vi "Gate Delay Control.vi"(7 "Calling VI Ref":refnum<vi>) -> ()   [LabVIEW 2016]
uses:
  Gate Delay Type Defs/Delay Control.ctl
  <vilib>/Utility/miscctls.llb/LVPointTypeDef.ctl
  <vilib>/event_ctls.llb/lveventtype.ctl
  Gate Delay Type Defs/Board Names.ctl
  Gate Delay Type Defs/Gate Delay Actions.ctl
panel:
  in  "Link":bool
  in  "Restore Defaults":bool
  in  "Set Defaults":bool
  in  "Board Selection":enum32{"Delay 01", "Delay 02"}(radio)
  in  "Window Width":T1 {"Delay Slider" scale=0.0..9.5; "Delay (ns)" format="%#_4g"}
  in  "Window Delay":T1 {"Delay Slider" scale=0.0..19.5; "Delay (ns)" format="%#_4g"}
  in  "Laser Delay":T1 {"Delay Slider" scale=0.0..19.5; "Delay (ns)" format="%#_4g"}
  in  "Quit":bool
  # "Delay (ns)"
  # "Step (ns)"
  # "Window Width"
  # "Window Delay"
  # "Laser Delay"
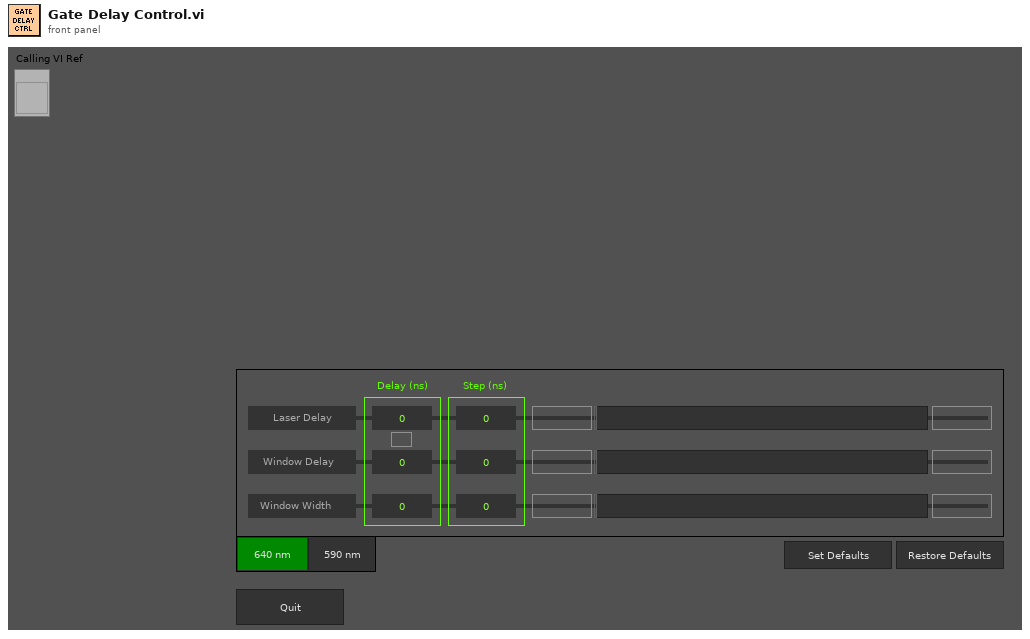
[diagram p1: front panel]
types:
  T1 = typedef "Delay Control.ctl" = cluster{"Delay (ns)":dbl, "Step (ns)":dbl, "Step Minus":bool, "Delay Slider":dbl, "Step Plus":bool}
  T2 = enum16{"Always On", "Always Off", "Off While Running"}
  T3 = typedef "LVPointTypeDef.ctl" = cluster{"Horizontal":i16, "Vertical":i16}
  T4 = typedef "lveventtype.ctl" = enum32{"Null", "Timeout", "Annotation Menu Selection", "Annotation Menu Selection?", "App Instance Close", "App Instance Close?", "Autoscale Range Change", "Bookmark Info Change", "Cell Edit", "Cell Edit?", "Cursor Grab", "Cursor Grab?", "Cursor Menu Selection", "Cursor Menu Selection?", "Cursor Move", "Cursor Release", "Data Change", "Direction Change", "Display State Change", "Drag Ended", "Drag Enter", "Drag Leave", "Drag Over", "Drag Source Update", "Drag Starting", "Drag Starting?", "Drop", "Exec State Change", "Key Down", "Key Down?", "Key Repeat", "Key Repeat?", "Key Up", "Listbox Double Click", "Menu Activation?", "Menu Selection (App)", "Menu Selection? (App)", "Menu Selection (User)", "Mouse Down", "Mouse Down?", "Mouse Enter", "Mouse Leave", "Mouse Move", "Mouse Up", "Mouse Wheel", "NI Security User Change (App)", "Pane Size", "Panel Close", "Panel Close?", "Panel Resize", "Plot Attribute Change", "Scale Range Change", "Shortcut Menu Activation?", "Shortcut Menu Selection (App)", "Shortcut Menu Selection? (App)", "Shortcut Menu Selection (User)", "Tree Double Click", "Tree Drag", "Tree Drag?", "Tree Drop", "Tree Drop?", "Tree Item Close", "Tree Item Close?", "Tree Item Open", "Tree Item Open?", "User Event", "Value Change"}
  T5 = typedef "Gate Delay Actions.ctl" = enum16{"Set Laser Delay", "Set Window Delay", "Set Window Width", "Get Delays", "Set Default Delays", "Restore Defaults", "Quit"}
  T6 = typedef "Board Names.ctl" = enum16{"Gate Delay 01", "Gate Delay 02"}
  T7 = enum32{"Bad", "Idle", "Run top level", "Running"}
  T8 = typedef "LVRectTypeDef.ctl" = cluster{"Left":i16, "Top":i16, "Right":i16, "Bottom":i16}
  T9 = typedef "LVBoundsTypeDef.ctl" = cluster{"Width":u32, "Height":u32}
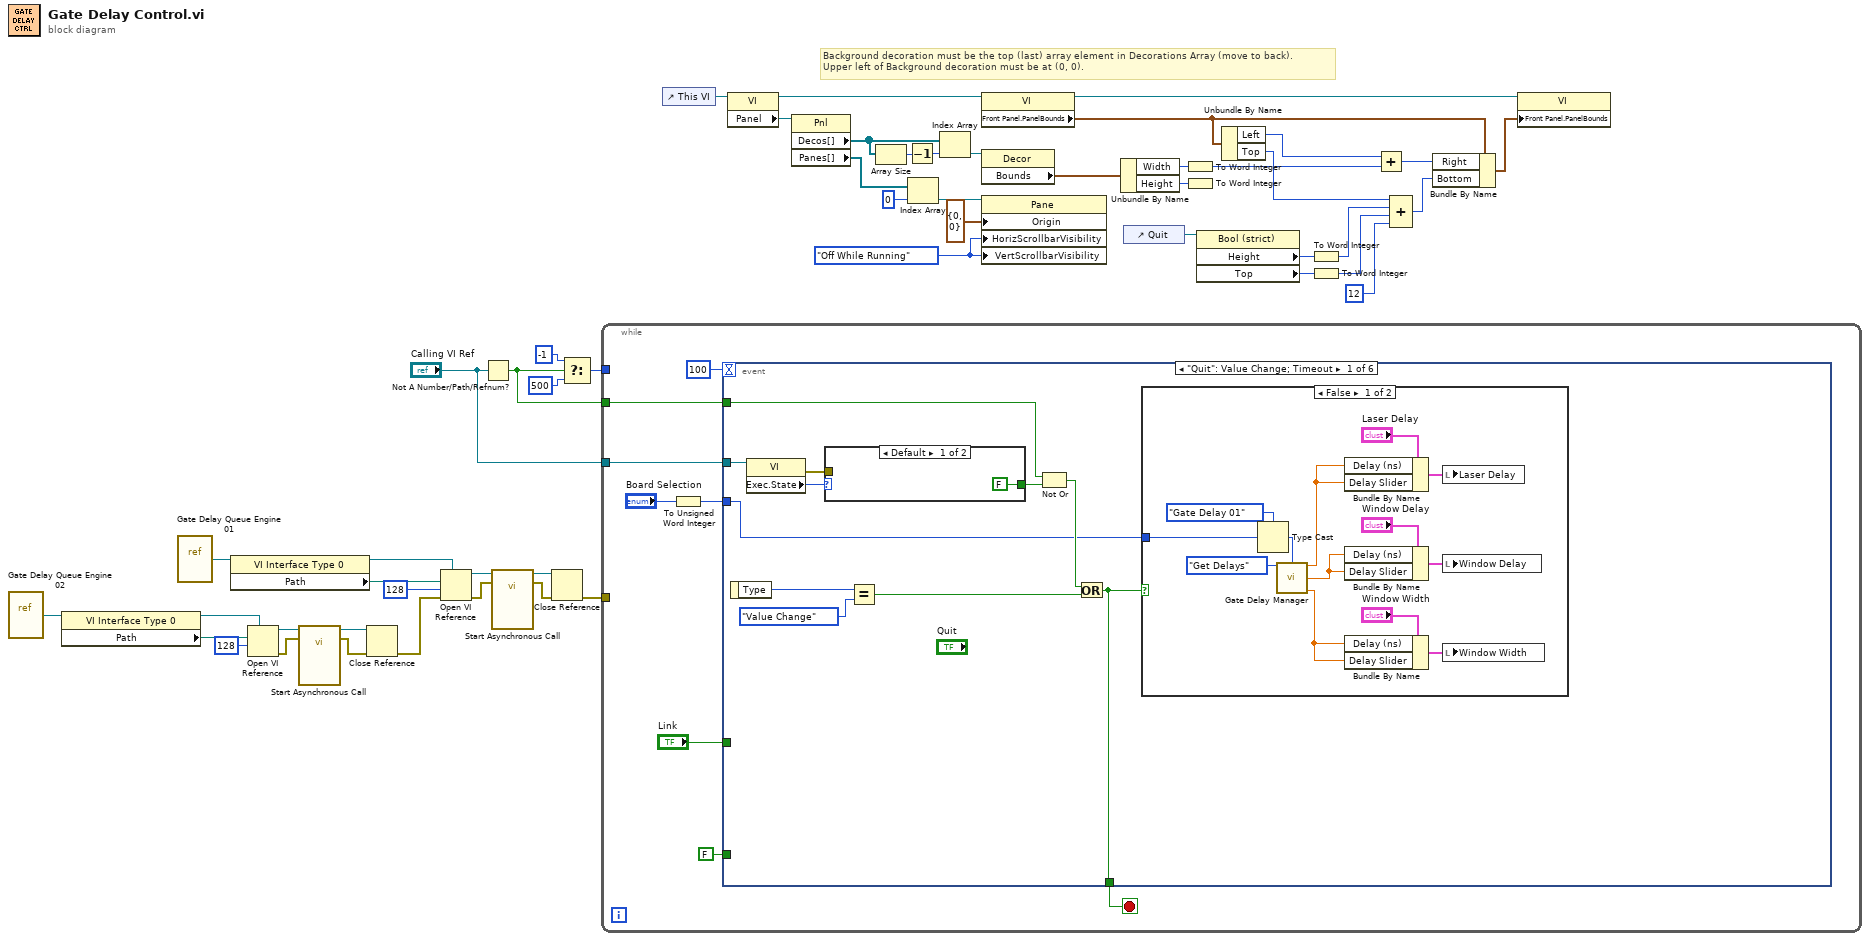
[diagram p0: block diagram]
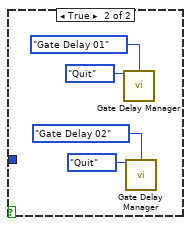
[diagram p2: hidden frame]
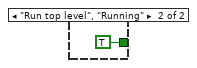
[diagram p3: hidden frame]
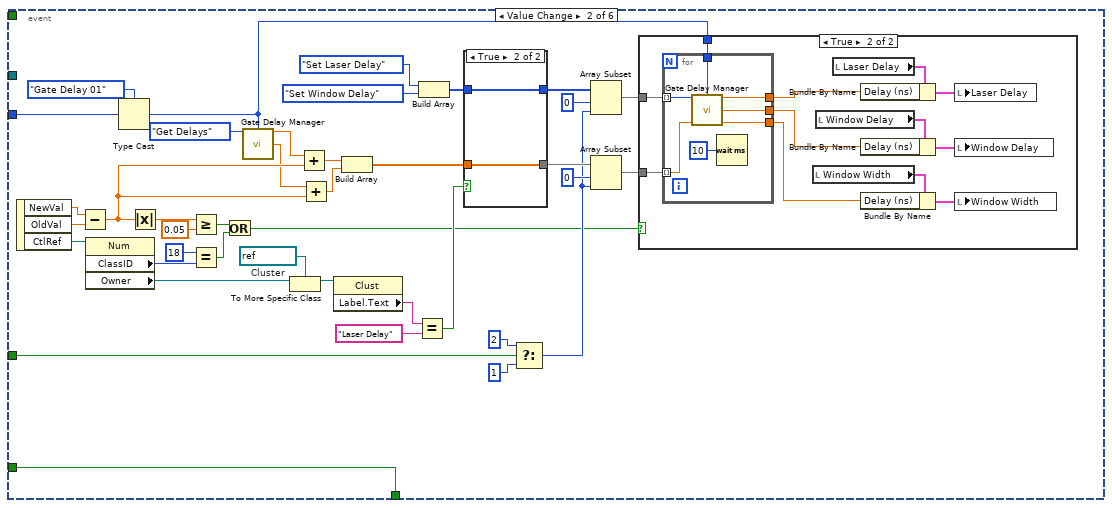
[diagram p4: hidden frame]
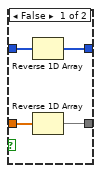
[diagram p6: hidden frame]
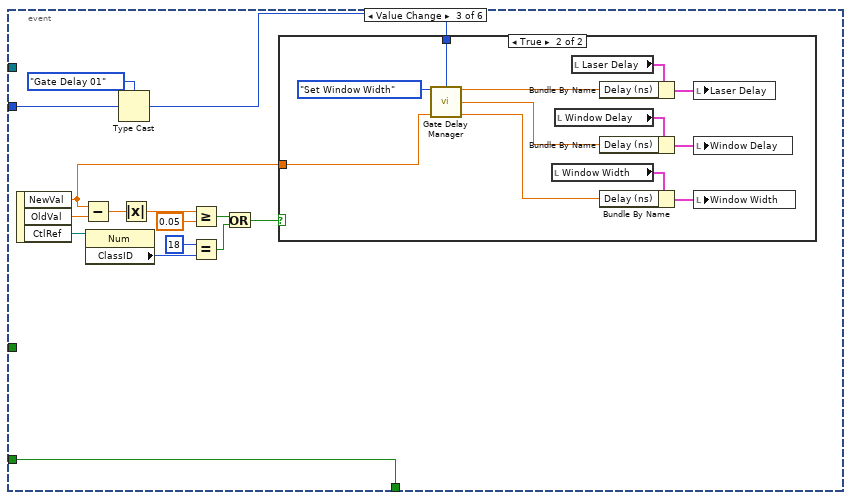
[diagram p7: hidden frame]
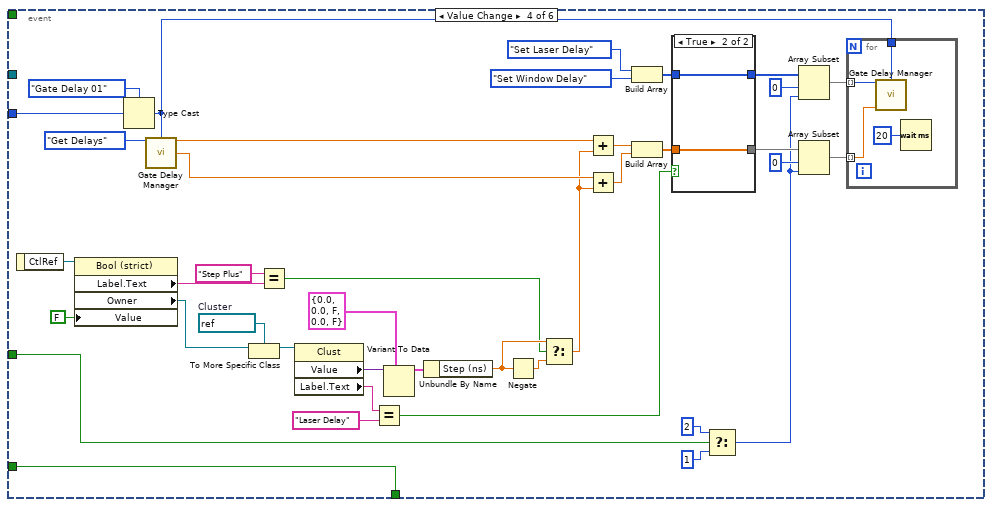
[diagram p9: hidden frame]
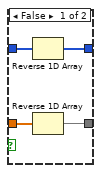
[diagram p10: hidden frame]
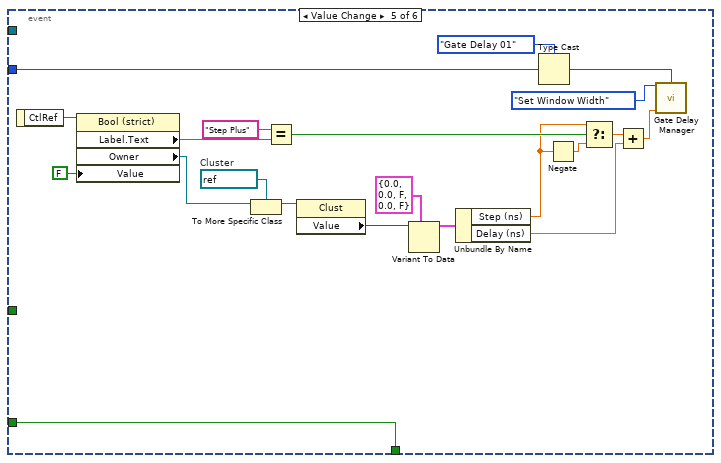
[diagram p11: hidden frame]
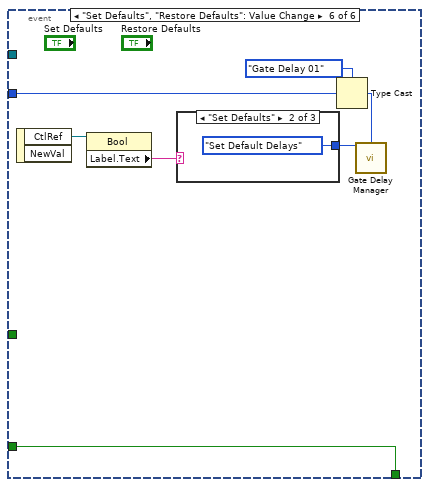
[diagram p12: hidden frame]
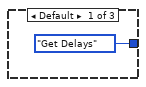
[diagram p13: hidden frame]
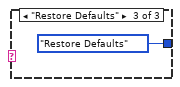
[diagram p14: hidden frame]
diagram:
  w30 = T2."Off While Running" ("Vertical Scrollbar Visibility")
  # "Background decoration must be the top (last) array element in Decorations Array (move to back).\nUpper left of Background decoration must be at (0, 0)."
  n1 = vi-ref "Gate Delay Queue Engine 02.vi"() -> (w11:refnum<vi>)
  n2 = property class="VI Interface Type 0"(reference=w11) -> (reference out=w9:refnum<vi>, "Path"=w10:path)  [unwired: 1 in, 1 out]
  n3 = vi-ref "Gate Delay Queue Engine 01.vi"() -> (w17:refnum<vi>)
  n4 = property class="VI Interface Type 0"(reference=w17) -> (reference out=w15:refnum<vi>, "Path"=w16:path)  [unwired: 1 in, 1 out]
  n5 = Open VI Reference(type specifier VI Refnum (for type only)=w9, vi path=w10, options=128) -> (vi reference=w8:refnum<vi>, error out=w6:errorcluster)  [unwired: 3 in]
  n6 = call-by-ref "Start Asynchronous Call"(reference=w8, error in=w6) -> (reference out=w7:refnum<vi>, error out=w5:errorcluster)  [unwired: 12 in]
  n7 = Close Reference(reference=w7, error in (no error)=w5) -> (error out=w4:errorcluster)
  n8 = Open VI Reference(type specifier VI Refnum (for type only)=w15, vi path=w16, options=128, error in (no error)=w4) -> (vi reference=w14:refnum<vi>, error out=w3:errorcluster)  [unwired: 2 in]
  n9 = Not A Number/Path/Refnum?(number/path/refnum="Calling VI Ref") -> (NaN/Path/Refnum?=w48:bool)
  n10 = call-by-ref "Start Asynchronous Call"(reference=w14, error in=w3) -> (reference out=w13:refnum<vi>, error out=w2:errorcluster)  [unwired: 12 in]
  n11 = Close Reference(reference=w13, error in (no error)=w2) -> (error out=w1:errorcluster)
  n12 = Select(t=-1, s=w48, f=500) -> (s? t:f=w50:i32)
  n13 = while {
    tunnel: w50 -> [_]
    tunnel: "Calling VI Ref" -> [w58]
    tunnel: w48 -> [w57]
    tunnel: w1 -> [_]
    stop <- w60 stop-if-true
    n14 = To Unsigned Word Integer(number="Board Selection") -> (unsigned 16bit integer=w55:u16)
    n15 = event shown="[0] \"Quit\": Value Change;  Timeout" {
      selector: _ -> [_ _ _ _ _ _]
      dyn-events: _ -> [_ _ _ _ _ _]
      timeout: 100 -> [_ _ _ _ _ _]
      tunnel: [w62 w130 w170 w222 w253 w260] -> w60
      tunnel: FALSE ("NewVal") -> [_ w130 w170 w222 w253 w260]
      tunnel: w58 -> [w71 _ _ _ _ _]
      tunnel: w57 -> [w66 _ _ _ _ _]
      tunnel: w55 -> [w61 w116 w160 w213 w240 w255]
      tunnel: "Link" -> [_ w100 _ w188 _ _]
      event "Quit": Value Change; Timeout {
        n16 = event-data() -> ("Type"=w69:T4)  [unwired: 1 in]
        n17 = property class="VI"(reference=w71) -> (error out=w63:errorcluster, "Exec.State"=w70:T7)  [unwired: 1 in, 1 out]
        n18 = case shown="Default" w70 {
          tunnel: [FALSE TRUE] -> w65
          tunnel: w63 -> [_ _]
          frame Default {
          }
          frame "Run top level", "Running" {
          }
        }
        n19 = Equal?(x=w69, y=lveventtype."Value Change" ("Type")) -> (x = y?=w67:bool)
        n20 = Not Or(1:w65, 2:w66) -> (0:w64:bool)
        n21 = Or(x=w64, y=w67) -> (x .or. y?=w62:bool)
        n22 = case shown="False" w62 {
          tunnel: w61 -> [w72 _]
          frame False {
            n23 = Type Cast(type=Board_Names."Gate Delay 01" ("Gate Delay Names"), x=w72) -> (*(type *) &x=w84:T6)
            n24 = call "Gate Delay Manager.vi"("Gate Delay Actions"=Gate_Delay_Actions."Get Delays", "Gate Delay Names"=w84) -> ("Laser Delay (ns)"=w74:dbl, "Window Delay (ns)"=w75:dbl, "Window Width (ns)"=w73:dbl)  [unwired: 11 in]
            n25 = Bundle By Name(cluster="Laser Delay", "Delay (ns)"=w74, "Delay Slider"=w74) -> (w79:T1)
            n26 = Bundle By Name(cluster="Window Delay", "Delay (ns)"=w75, "Delay Slider"=w75) -> (w80:T1)
            n27 = Bundle By Name(cluster="Window Width", "Delay (ns)"=w73, "Delay Slider"=w73) -> (w81:T1)
            n28 = local write "Laser Delay"(w79) -> ()
            n29 = local write "Window Delay"(w80) -> ()
            n30 = local write "Window Width"(w81) -> ()
          }
          frame True {
            n31 = call "Gate Delay Manager.vi"("Gate Delay Actions"=Gate_Delay_Actions."Quit", "Gate Delay Names"=Board_Names."Gate Delay 01") -> ()  [unwired: 11 in, 3 out]
            n32 = call "Gate Delay Manager.vi"("Gate Delay Actions"=Gate_Delay_Actions."Quit", "Gate Delay Names"=Board_Names."Gate Delay 02") -> ()  [unwired: 11 in, 3 out]
          }
        }
      }
      event Value Change {
        w120 = refnum<vi> refnum  # Cluster
        n33 = event-data() -> ("NewVal"=w121:dbl, "OldVal"=w128:dbl, "CtlRef"=w129:refnum<vi>)  [unwired: 1 in]
        n34 = Subtract(x=w121, y=w128) -> (x-y=w110:dbl)
        n35 = property class="Num"(reference=w129) -> ("ClassID"=w122:u32, "Owner"=w118:refnum<vi>)  [unwired: 1 in, 2 out]
        n36 = Type Cast(type=Board_Names."Gate Delay 01" ("Gate Delay Names"), x=w116) -> (*(type *) &x=w94:T6)
        n37 = Absolute Value(x=w110) -> (abs(x)=w127:dbl)
        n38 = Greater Or Equal?(x=w127, y=0.05) -> (x >= y?=w125:bool)
        n39 = Equal?(x=u32 18 ("y"), y=w122) -> (x = y?=w124:bool)
        n40 = Or(x=w125, y=w124) -> (x .or. y?=w91:bool)
        n41 = call "Gate Delay Manager.vi"("Gate Delay Actions"=Gate_Delay_Actions."Get Delays", "Gate Delay Names"=w94) -> ("Laser Delay (ns)"=w108:dbl, "Window Delay (ns)"=w109:dbl)  [unwired: 11 in, 1 out]
        n42 = To More Specific Class(target class=w120, reference=w118) -> (specific class reference=w119:refnum<vi>)  [unwired: 1 in, 1 out]
        n43 = Add(x=w108, y=w110) -> (x+y=w107:dbl)
        n44 = Add(x=w109, y=w110) -> (x+y=w106:dbl)
        n45 = property class="Clust"(reference=w119) -> ("Label.Text"=w112:string)  [unwired: 1 in, 2 out]
        n46 = Build Array(w107, w106) -> (w104:dbl[])
        n47 = Equal?(x=w112, y="Laser Delay") -> (x = y?=w103:bool)
        n48 = Build Array(Gate_Delay_Actions."Set Laser Delay" ("Gate Delay Actions"), Gate_Delay_Actions."Set Window Delay" ("Gate Delay Actions")) -> (w105:T5[])
        n49 = case shown="True" w103 {
          tunnel: w105 -> [w153 w155]
          tunnel: w104 -> [w152 w154]
          tunnel: [w151 w155] -> w102
          tunnel: [w150 w154] -> w101
          frame False {
            n50 = Reverse 1D Array(array=w153) -> (reversed array=w151:T5[])
            n51 = Reverse 1D Array(array=w152) -> (reversed array=w150:dbl[])
          }
          frame True {
          }
        }
        n52 = Select(t=2 ("index"), s=w100, f=1 ("index")) -> (s? t:f=w95:i32)
        n53 = Array Subset(array=w102, index=0, length=w95) -> (w93:T5[])
        n54 = Array Subset(array=w101, index=0, length=w95) -> (w92:dbl[])
        n55 = case shown="True" w91 {
          tunnel: w94 -> [_ w140]
          tunnel: w93 -> [_ w142]
          tunnel: w92 -> [_ w141]
          frame False {
          }
          frame True {
            n56 = for {
              tunnel: w142 -> [w148] mode=indexing
              tunnel: w141 -> [w147] mode=indexing
              tunnel: w140 -> [w149]
              tunnel: [w145] -> w133
              tunnel: [w144] -> w132
              tunnel: [w143] -> w131
              n57 = call "Gate Delay Manager.vi"("Gate Delay Actions"=w148, "Gate Delay Names"=w149, "Delay Time In (ns)"=w147) -> ("Laser Delay (ns)"=w145:dbl, "Window Delay (ns)"=w144:dbl, "Window Width (ns)"=w143:dbl)  [unwired: 10 in]
              n58 = Wait (ms)(milliseconds to wait=u32 10) -> ()  [unwired: 1 out]
            }
            n59 = local read "Window Width"() -> (w134:T1)
            n60 = local read "Window Delay"() -> (w135:T1)
            n61 = local read "Laser Delay"() -> (w136:T1)
            n62 = Bundle By Name(cluster=w136, "Delay (ns)"=w133) -> (w139:T1)
            n63 = Bundle By Name(cluster=w135, "Delay (ns)"=w132) -> (w138:T1)
            n64 = Bundle By Name(cluster=w134, "Delay (ns)"=w131) -> (w137:T1)
            n65 = local write "Laser Delay"(w139) -> ()
            n66 = local write "Window Delay"(w138) -> ()
            n67 = local write "Window Width"(w137) -> ()
          }
        }
      }
      event Value Change {
        n68 = event-data() -> ("NewVal"=w156:dbl, "OldVal"=w168:dbl, "CtlRef"=w169:refnum<vi>)  [unwired: 1 in]
        n69 = Subtract(x=w156, y=w168) -> (x-y=w157:dbl)
        n70 = property class="Num"(reference=w169) -> ("ClassID"=w162:u32)  [unwired: 1 in, 2 out]
        n71 = Type Cast(type=Board_Names."Gate Delay 01" ("Gate Delay Names"), x=w160) -> (*(type *) &x=w159:T6)
        n72 = Absolute Value(x=w157) -> (abs(x)=w167:dbl)
        n73 = Greater Or Equal?(x=w167, y=0.05) -> (x >= y?=w165:bool)
        n74 = Equal?(x=u32 18 ("y"), y=w162) -> (x = y?=w164:bool)
        n75 = Or(x=w165, y=w164) -> (x .or. y?=w158:bool)
        n76 = case shown="True" w158 {
          tunnel: w159 -> [_ w181]
          tunnel: w156 -> [_ w182]
          frame False {
          }
          frame True {
            n77 = call "Gate Delay Manager.vi"("Gate Delay Actions"=Gate_Delay_Actions."Set Window Width", "Gate Delay Names"=w181, "Delay Time In (ns)"=w182) -> ("Laser Delay (ns)"=w174:dbl, "Window Delay (ns)"=w173:dbl, "Window Width (ns)"=w172:dbl)  [unwired: 10 in]
            n78 = local read "Window Width"() -> (w175:T1)
            n79 = local read "Window Delay"() -> (w176:T1)
            n80 = local read "Laser Delay"() -> (w177:T1)
            n81 = Bundle By Name(cluster=w177, "Delay (ns)"=w174) -> (w180:T1)
            n82 = Bundle By Name(cluster=w176, "Delay (ns)"=w173) -> (w179:T1)
            n83 = Bundle By Name(cluster=w175, "Delay (ns)"=w172) -> (w178:T1)
            n84 = local write "Laser Delay"(w180) -> ()
            n85 = local write "Window Delay"(w179) -> ()
            n86 = local write "Window Width"(w178) -> ()
          }
        }
      }
      event Value Change {
        w220 = refnum<vi> refnum  # Cluster
        n87 = event-data() -> ("CtlRef"=w221:refnum<vi>)  [unwired: 1 in]
        n88 = property class="Bool (strict)"(reference=w221, "Value"=FALSE) -> ("Label.Text"=w216:string, "Owner"=w218:refnum<vi>)  [unwired: 1 in, 2 out]
        n89 = Type Cast(type=Board_Names."Gate Delay 01" ("Gate Delay Names"), x=w213) -> (*(type *) &x=w184:T6)
        n90 = call "Gate Delay Manager.vi"("Gate Delay Actions"=Gate_Delay_Actions."Get Delays", "Gate Delay Names"=w184) -> ("Laser Delay (ns)"=w205:dbl, "Window Delay (ns)"=w204:dbl)  [unwired: 11 in, 1 out]
        n91 = To More Specific Class(target class=w220, reference=w218) -> (specific class reference=w219:refnum<vi>)  [unwired: 1 in, 1 out]
        n92 = Equal?(x="Step Plus", y=w216) -> (x = y?=w206:bool)
        n93 = property class="Clust"(reference=w219) -> ("Value"=w207:variant, "Label.Text"=w193:string)  [unwired: 1 in, 2 out]
        n94 = Equal?(x=w193, y="Laser Delay") -> (x = y?=w192:bool)
        n95 = Variant To Data(type=T1 {"Delay (ns)"=0.0, "Step (ns)"=0.0, "Step Minus"=FALSE, "Delay Slider"=0.0, "Step Plus"=FALSE} ("Delay Control"), Variant=w207) -> (data=w210:T1)  [unwired: 1 in, 1 out]
        n96 = Unbundle By Name(w210) -> ("Step (ns)"=w214:dbl)
        n97 = Negate(x=w214) -> (-x=w212:dbl)
        n98 = Select(t=w214, s=w206, f=w212) -> (s? t:f=w203:dbl)
        n99 = Add(x=w205, y=w203) -> (x+y=w194:dbl)
        n100 = Add(x=w204, y=w203) -> (x+y=w191:dbl)
        n101 = Build Array(Gate_Delay_Actions."Set Laser Delay" ("Gate Delay Actions"), Gate_Delay_Actions."Set Window Delay" ("Gate Delay Actions")) -> (w200:T5[])
        n102 = Build Array(w194, w191) -> (w199:dbl[])
        n103 = case shown="True" w192 {
          tunnel: w200 -> [w230 w232]
          tunnel: w199 -> [w229 w231]
          tunnel: [w228 w232] -> w198
          tunnel: [w227 w231] -> w197
          frame False {
            n104 = Reverse 1D Array(array=w230) -> (reversed array=w228:T5[])
            n105 = Reverse 1D Array(array=w229) -> (reversed array=w227:dbl[])
          }
          frame True {
          }
        }
        n106 = Select(t=2 ("index"), s=w188, f=1 ("index")) -> (s? t:f=w187:i32)
        n107 = Array Subset(array=w198, index=0, length=w187) -> (w186:T5[])
        n108 = Array Subset(array=w197, index=0, length=w187) -> (w185:dbl[])
        n109 = for {
          tunnel: w186 -> [w225] mode=indexing
          tunnel: w185 -> [w224] mode=indexing
          tunnel: w184 -> [w226]
          n110 = call "Gate Delay Manager.vi"("Gate Delay Actions"=w225, "Gate Delay Names"=w226, "Delay Time In (ns)"=w224) -> ()  [unwired: 10 in, 3 out]
          n111 = Wait (ms)(milliseconds to wait=u32 20) -> ()  [unwired: 1 out]
        }
      }
      event Value Change {
        w251 = refnum<vi> refnum  # Cluster
        n112 = event-data() -> ("CtlRef"=w252:refnum<vi>)  [unwired: 1 in]
        n113 = property class="Bool (strict)"(reference=w252, "Value"=FALSE) -> ("Label.Text"=w245:string, "Owner"=w249:refnum<vi>)  [unwired: 1 in, 2 out]
        n114 = To More Specific Class(target class=w251, reference=w249) -> (specific class reference=w250:refnum<vi>)  [unwired: 1 in, 1 out]
        n115 = Equal?(x="Step Plus", y=w245) -> (x = y?=w243:bool)
        n116 = property class="Clust"(reference=w250) -> ("Value"=w248:variant)  [unwired: 1 in, 2 out]
        n117 = Variant To Data(type=T1 {"Delay (ns)"=0.0, "Step (ns)"=0.0, "Step Minus"=FALSE, "Delay Slider"=0.0, "Step Plus"=FALSE} ("Delay Control"), Variant=w248) -> (data=w246:T1)  [unwired: 1 in, 1 out]
        n118 = Unbundle By Name(w246) -> ("Step (ns)"=w242:dbl, "Delay (ns)"=w241:dbl)
        n119 = Type Cast(type=Board_Names."Gate Delay 01" ("Gate Delay Names"), x=w240) -> (*(type *) &x=w237:T6)
        n120 = Negate(x=w242) -> (-x=w239:dbl)
        n121 = Select(t=w242, s=w243, f=w239) -> (s? t:f=w238:dbl)
        n122 = Add(x=w238, y=w241) -> (x+y=w235:dbl)
        n123 = call "Gate Delay Manager.vi"("Gate Delay Actions"=Gate_Delay_Actions."Set Window Width", "Gate Delay Names"=w237, "Delay Time In (ns)"=w235) -> ()  [unwired: 10 in, 3 out]
      }
      event "Set Defaults", "Restore Defaults": Value Change {
        n124 = event-data() -> ("CtlRef"=w259:refnum<vi>)  [unwired: 1 in, 1 out]
        n125 = property class="Bool"(reference=w259) -> ("Label.Text"=w258:string)  [unwired: 1 in, 2 out]
        n126 = case shown="\"Set Defaults\"" w258 {
          tunnel: [Gate_Delay_Actions."Get Delays" ("Gate Delay Actions") Gate_Delay_Actions."Set Default Delays" ("Gate Delay Actions") Gate_Delay_Actions."Restore Defaults" ("Gate Delay Actions")] -> w254
          frame Default {
          }
          frame "Set Defaults" {
          }
          frame "Restore Defaults" {
          }
        }
        n127 = Type Cast(type=Board_Names."Gate Delay 01" ("Gate Delay Names"), x=w255) -> (*(type *) &x=w257:T6)
        n128 = call "Gate Delay Manager.vi"("Gate Delay Actions"=w254, "Gate Delay Names"=w257) -> ()  [unwired: 11 in, 3 out]
      }
    }
  }
  n129 = control-ref of="This VI"() -> (w22:refnum<vi>)
  n130 = property class="VI"(reference=w22) -> (reference out=w31:refnum<vi>, "Panel"=w23:refnum<vi>)  [unwired: 1 in, 1 out]
  n131 = property class="Pnl"(reference=w23) -> ("Decos[]"=w21:refnum<vi>[], "Panes[]"=w27:refnum<vi>[])  [unwired: 1 in, 2 out]
  n132 = Array Size(array=w21) -> (size(s)=w19:i32)
  n133 = Decrement(x=w19) -> (x-1=w20:i32)
  n134 = Index Array(array=w27, index=0) -> (element=w26:refnum<vi>)
  n135 = Index Array(array=w21, index=w20) -> (element=w29:refnum<vi>)
  n136 = property class="VI"(reference=w31) -> (reference out=w33:refnum<vi>, "Front Panel.PanelBounds"=w34:T8)  [unwired: 1 in, 1 out]
  n137 = property class="Decor"(reference=w29) -> ("Bounds"=w32:T9)  [unwired: 1 in, 2 out]
  n138 = property class="Pane"(reference=w26, "Origin"=T3 {"Horizontal"=0, "Vertical"=0}, "HorizScrollbarVisibility"=w30, "VertScrollbarVisibility"=w30) -> ()  [unwired: 1 in, 2 out]
  n139 = Unbundle By Name(w32) -> ("Width"=w37:u32, "Height"=w40:u32)
  n140 = control-ref of="Quit"() -> (w24:refnum<vi>)
  n141 = To Word Integer(number=w37) -> (16bit integer=w39:i16)
  n142 = To Word Integer(number=w40) -> ()  [unwired: 1 out]
  n143 = property class="Bool (strict)"(reference=w24) -> ("Height"=w42:u32, "Top"=w43:i32)  [unwired: 1 in, 2 out]
  n144 = Unbundle By Name(w34) -> ("Left"=w36:i16, "Top"=w47:i16)
  n145 = To Word Integer(number=w42) -> (16bit integer=w45:i16)
  n146 = To Word Integer(number=w43) -> (16bit integer=w46:i16)
  n147 = Add(x=w36, y=w39) -> (x+y=w38:i16)
  n148 = Compound Arithmetic op=ADD(w47, w45, w46, i16 12 ("y")) -> (w41:i16)
  n149 = Bundle By Name(cluster=w34, "Right"=w38, "Bottom"=w41) -> (w35:T8)
  n150 = property class="VI"(reference=w33, "Front Panel.PanelBounds"=w35) -> ()  [unwired: 1 in, 2 out]
